vi "Read directory.vi"(8 "error in (no error)":errorcluster, 11 "Log File in":refnum<class "CM_Log File.lvclass">) -> (0 "error out":errorcluster, 2 "directory":path, 3 "Log File out":refnum<class "CM_Log File.lvclass">)   [LabVIEW 2018, in "CM_Log File.lvclass"]
uses:
  CM_Log File.lvclass
  CM_Log File.lvclass/CM_Log File.ctl
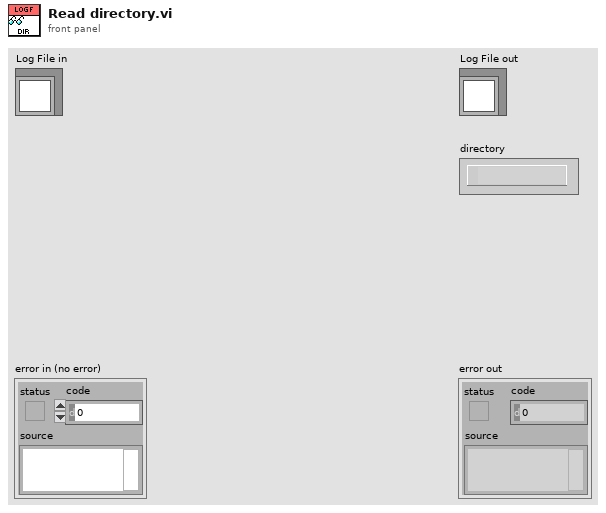
[diagram p1: front panel]
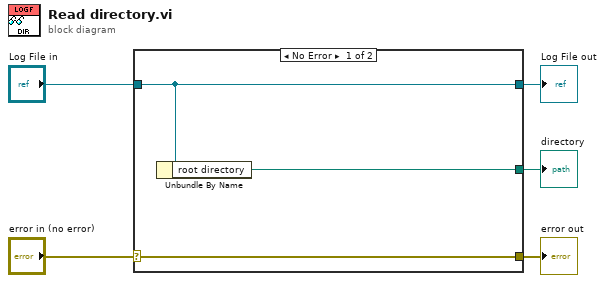
[diagram p0: block diagram]
diagram:
  n1 = case shown="No Error" "error in (no error)" {
    selector: "error in (no error)" -> [w8 w9]
    tunnel: [w8 w9] -> w4
    tunnel: [w7 w10] -> w2
    tunnel: "Log File in" -> [w7 w10]
    tunnel: [w6 _] -> w1
    frame No Error {
      n2 = Unbundle By Name(w7) -> ("root directory"=w6:path)
    }
    frame Error {
    }
  }
  "error out" <- w4
  "Log File out" <- w2
  "directory" <- w1
